vi "test-leadLag-test1.vi"(8 "error in (no error)":errorcluster) -> (0 "error out":errorcluster, 3 "All  PASSED":bool)   [LabVIEW 2019]
uses:
  <vilib>/Rock Robotics/WPI/ThirdParty/JAS_Junk/TrajLib/Util_GetTime.vi
  <vilib>/Rock Robotics/WPI/ThirdParty/JAS_Junk/TrajLib/Trajectory_Library.lvlib
panel:
  out "Lag Test Passed 2":bool
  out "Lag Chart 2":cluster{"Output":dbl, dbl}(graph)
  out "Lead Lag Test Passed":bool
  out "Lead Lag Chart":cluster{"Output":dbl, dbl}(graph)
  out "Lead Test Passed":bool
  out "Lead Test Chart":cluster{"Output":dbl, dbl}(graph)
  out "Test No Lead or Lag":bool
  out "Test No Lead or Lag":cluster{"Output":dbl, dbl}(graph)
  out "Lag Test Passed":bool
  out "Lag Chart":cluster{"Output":dbl, dbl}(graph)
  # "NOT A TEST....."
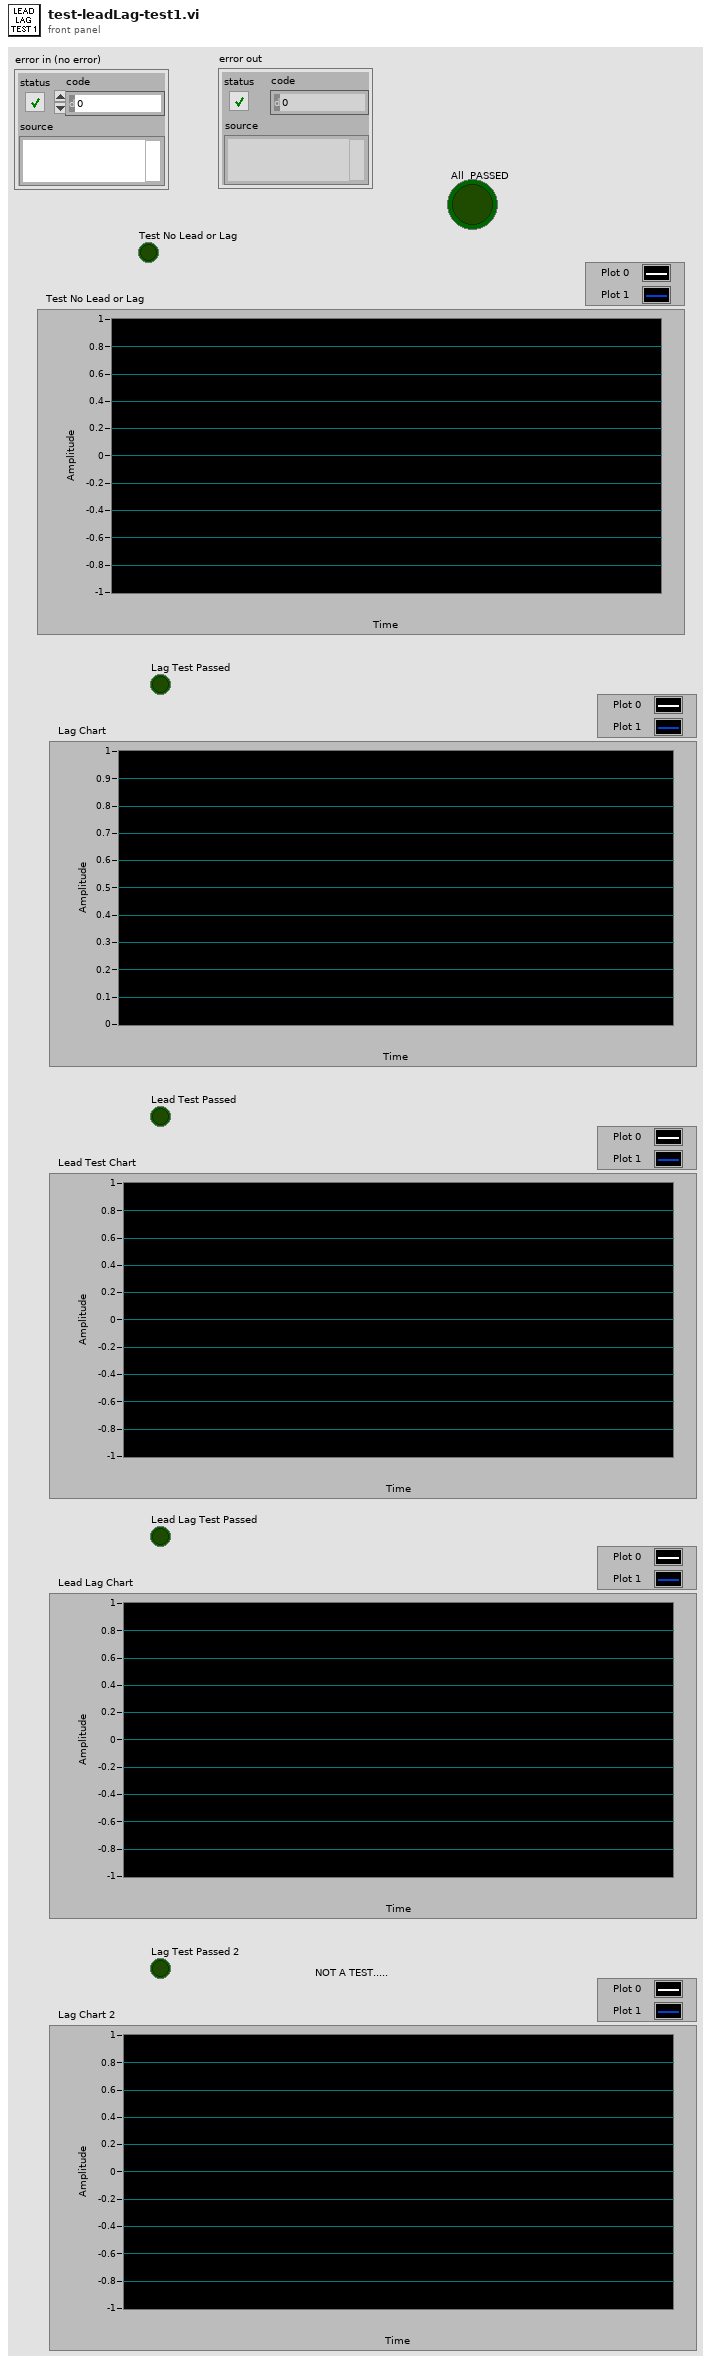
[diagram p1: front panel]
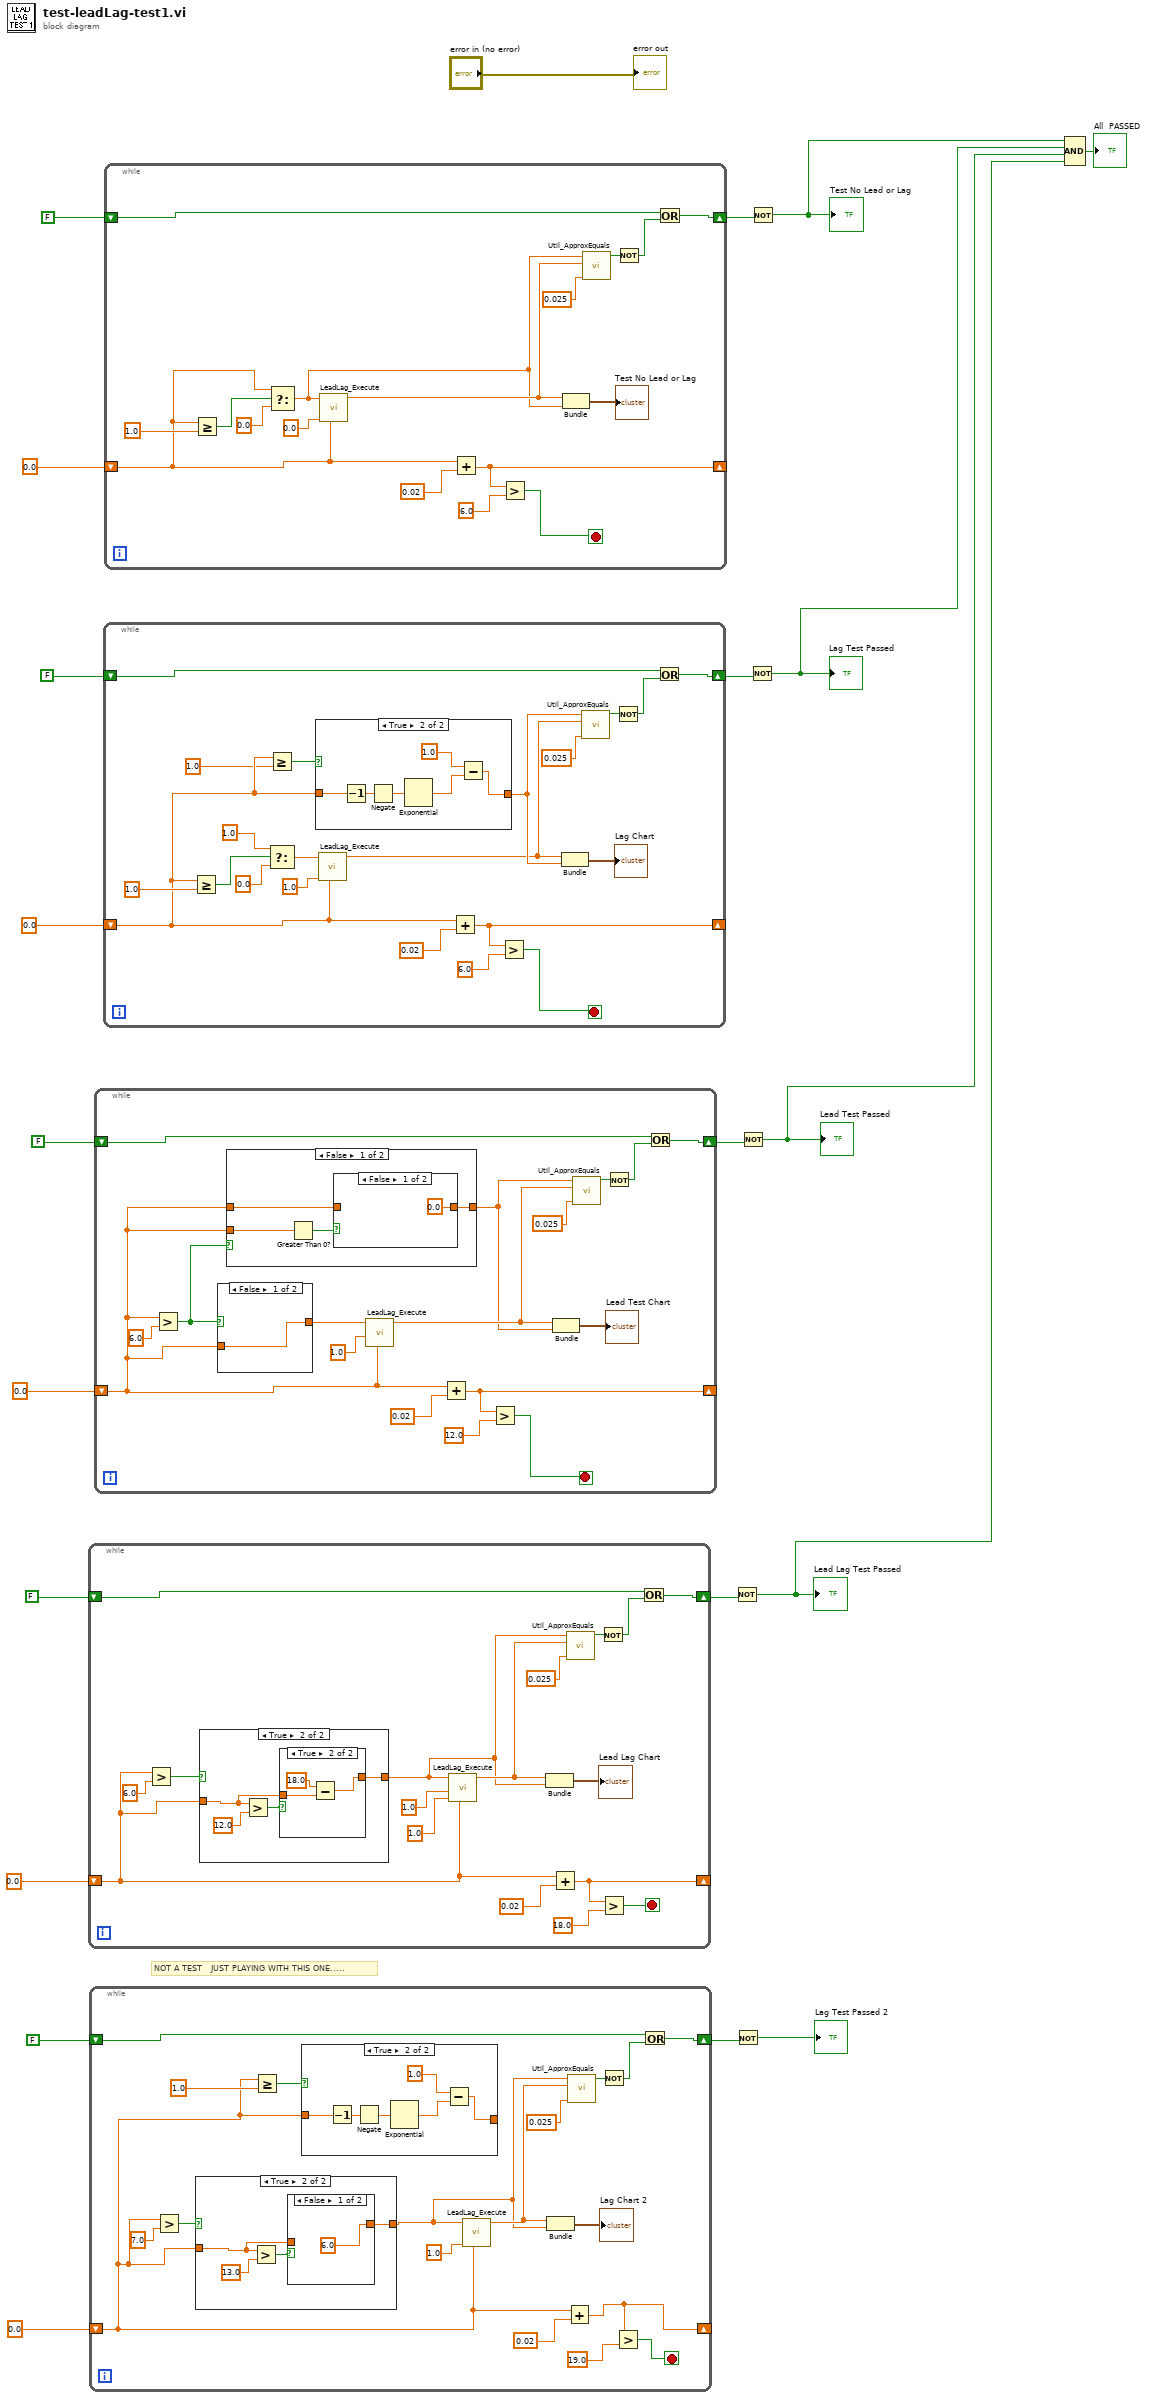
[diagram p0: block diagram]
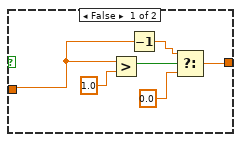
[diagram p2: hidden frame]
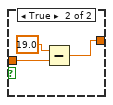
[diagram p3: hidden frame]
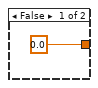
[diagram p4: hidden frame]
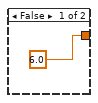
[diagram p6: hidden frame]
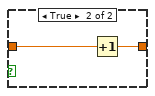
[diagram p7: hidden frame]
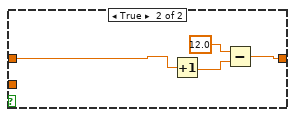
[diagram p8: hidden frame]
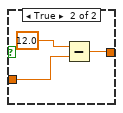
[diagram p9: hidden frame]
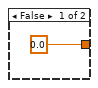
[diagram p10: hidden frame]
diagram:
  # "NOT A TEST   JUST PLAYING WITH THIS ONE....."
  n1 = while {
    shift-right: [w38] -> _
    shift-left: 0.0 -> [w27]
    shift-right: [w31] -> w11
    shift-left: FALSE -> [w33]
    stop <- w36 stop-if-true
    n2 = Greater?(x=w27, y=6.0) -> (0:w28:bool)
    n3 = case shown="True" w28 {
      tunnel: [w40 w42] -> w23
      tunnel: w27 -> [w40 w41]
      frame False {
      }
      frame True {
        n4 = Greater?(x=w41, y=12.0) -> (0:w43:bool)
        n5 = case shown="True" w43 {
          tunnel: [6.0 w48] -> w42
          tunnel: w41 -> [_ w46]
          frame False {
          }
          frame True {
            n6 = Subtract(x=18.0, y=w46) -> (x-y=w48:dbl)
          }
        }
      }
    }
    n7 = call <vilib>:"LeadLag_Execute.vi"("Time (Secs)"=w27, "Lag Time Const (Sec)"=1.0, "Lead Time Const (Sec)"=1.0 ("Lag Time Const (Sec)"), "Input"=w23) -> ("Output"=w29:dbl)  [unwired: 7 in]
    n8 = Bundle("Output"=w29, w23) -> (→"Lead Lag Chart":cluster{"Output":dbl, dbl})  [unwired: 1 in]
    n9 = Add(x=w27, y=0.02) -> (x+y=w38:dbl)
    n10 = call <vilib>:"Util_ApproxEquals.vi"("Tolerance"=0.025, "Value 2"=w29, "Value 1"=w23) -> ("ApproxEquals"=w34:bool)  [unwired: 8 in]
    n11 = Not(x=w34) -> (.not. x?=w32:bool)
    n12 = Greater?(x=w38, y=18.0) -> (0:w36:bool)
    n13 = Or(x=w33, y=w32) -> (x .or. y?=w31:bool)
  }
  n14 = while {
    shift-right: [w64] -> _
    shift-left: 0.0 -> [w50]
    shift-right: [w53] -> w8
    shift-left: FALSE -> [w55]
    stop <- w62 stop-if-true
    n15 = Greater?(x=w50, y=7.0) -> (0:w51:bool)
    n16 = case shown="True" w51 {
      tunnel: [w72 w74] -> w49
      tunnel: w50 -> [w67 w73]
      frame False {
        n17 = Greater?(x=w67, y=1.0) -> (0:w70:bool)
        n18 = Decrement(x=w67) -> (x-1=w68:dbl)
        n19 = Select(t=w68, s=w70, f=0.0) -> (s? t:f=w72:dbl)
      }
      frame True {
        n20 = Greater?(x=w73, y=13.0) -> (0:w75:bool)
        n21 = case shown="False" w75 {
          tunnel: [6.0 w80] -> w74
          tunnel: w73 -> [_ w78]
          frame False {
          }
          frame True {
            n22 = Subtract(x=19.0, y=w78) -> (x-y=w80:dbl)
          }
        }
      }
    }
    n23 = Greater Or Equal?(x=w50, y=1.0) -> (x >= y?=w61:bool)
    n24 = case shown="True" w61 {
      tunnel: w50 -> [_ w87]
      tunnel: [0.0 w82] -> _
      frame False {
      }
      frame True {
        n25 = Decrement(x=w87) -> (x-1=w85:dbl)
        n26 = Negate(x=w85) -> (-x=w84:dbl)
        n27 = Exponential(1:w84) -> (0:w83:dbl)
        n28 = Subtract(x=1.0, y=w83) -> (x-y=w82:dbl)
      }
    }
    n29 = call <vilib>:"LeadLag_Execute.vi"("Time (Secs)"=w50, "Lag Time Const (Sec)"=1.0, "Input"=w49) -> ("Output"=w58:dbl)  [unwired: 8 in]
    n30 = Bundle("Output"=w58, "f"=w49) -> (→"Lag Chart 2":cluster{"Output":dbl, "f":dbl})  [unwired: 1 in]
    n31 = Add(x=w50, y=0.02) -> (x+y=w64:dbl)
    n32 = call <vilib>:"Util_ApproxEquals.vi"("Tolerance"=0.025, "Value 2"=w58, "Value 1"=w49) -> ("ApproxEquals"=w56:bool)  [unwired: 8 in]
    n33 = Not(x=w56) -> (.not. x?=w54:bool)
    n34 = Greater?(x=w64, y=19.0) -> (0:w62:bool)
    n35 = Or(x=w55, y=w54) -> (x .or. y?=w53:bool)
  }
  n36 = while {
    shift-right: [w103] -> _
    shift-left: 0.0 -> [w88]
    shift-right: [w96] -> w14
    shift-left: FALSE -> [w98]
    stop <- w101 stop-if-true
    n37 = Greater?(x=w88, y=6.0) -> (0:w91:bool)
    n38 = case shown="False" w91 {
      tunnel: [w116 w119] -> w93
      tunnel: w88 -> [w116 w118]
      frame False {
      }
      frame True {
        n39 = Subtract(x=12.0, y=w118) -> (x-y=w119:dbl)
      }
    }
    n40 = case shown="False" w91 {
      tunnel: w88 -> [w108 w113]
      tunnel: [w107 w114] -> w90
      tunnel: w88 -> [w105 _]
      frame False {
        n41 = Greater Than 0?(x=w105) -> (x > 0?=w106:bool)
        n42 = case shown="False" w106 {
          tunnel: w108 -> [_ w111]
          tunnel: [0.0 w110] -> w107
          frame False {
          }
          frame True {
            n43 = Increment(x=w111) -> (x+1=w110:dbl)
          }
        }
      }
      frame True {
        n44 = Increment(x=w113) -> (x+1=w112:dbl)
        n45 = Subtract(x=12.0, y=w112) -> (x-y=w114:dbl)
      }
    }
    n46 = call <vilib>:"LeadLag_Execute.vi"("Time (Secs)"=w88, "Lead Time Const (Sec)"=1.0 ("Lag Time Const (Sec)"), "Input"=w93) -> ("Output"=w92:dbl)  [unwired: 8 in]
    n47 = Add(x=w88, y=0.02) -> (x+y=w103:dbl)
    n48 = Greater?(x=w103, y=12.0) -> (0:w101:bool)
    n49 = Bundle("Output"=w92, w90) -> (→"Lead Test Chart":cluster{"Output":dbl, dbl})  [unwired: 1 in]
    n50 = call <vilib>:"Util_ApproxEquals.vi"("Tolerance"=0.025, "Value 2"=w92, "Value 1"=w90) -> ("ApproxEquals"=w99:bool)  [unwired: 8 in]
    n51 = Not(x=w99) -> (.not. x?=w97:bool)
    n52 = Or(x=w98, y=w97) -> (x .or. y?=w96:bool)
  }
  n53 = while {
    shift-right: [w134] -> _
    shift-left: 0.0 -> [w128]
    shift-right: [w120] -> w20
    shift-left: FALSE -> [w122]
    stop <- w132 stop-if-true
    n54 = Greater Or Equal?(x=w128, y=1.0) -> (x >= y?=w138:bool)
    n55 = Greater Or Equal?(x=w128, y=1.0) -> (x >= y?=w131:bool)
    n56 = Select(t=1.0, s=w138, f=0.0) -> (s? t:f=w130:dbl)
    n57 = case shown="True" w131 {
      tunnel: w128 -> [_ w147]
      tunnel: [0.0 w142] -> w126
      frame False {
      }
      frame True {
        n58 = Decrement(x=w147) -> (x-1=w145:dbl)
        n59 = Negate(x=w145) -> (-x=w144:dbl)
        n60 = Exponential(1:w144) -> (0:w143:dbl)
        n61 = Subtract(x=1.0, y=w143) -> (x-y=w142:dbl)
      }
    }
    n62 = call <vilib>:"LeadLag_Execute.vi"("Time (Secs)"=w128, "Lag Time Const (Sec)"=1.0, "Input"=w130) -> ("Output"=w125:dbl)  [unwired: 8 in]
    n63 = Add(x=w128, y=0.02) -> (x+y=w134:dbl)
    n64 = Greater?(x=w134, y=6.0) -> (0:w132:bool)
    n65 = Bundle("Output"=w125, w126) -> (→"Lag Chart":cluster{"Output":dbl, dbl})  [unwired: 1 in]
    n66 = call <vilib>:"Util_ApproxEquals.vi"("Tolerance"=0.025, "Value 2"=w125, "Value 1"=w126) -> ("ApproxEquals"=w123:bool)  [unwired: 8 in]
    n67 = Not(x=w123) -> (.not. x?=w121:bool)
    n68 = Or(x=w122, y=w121) -> (x .or. y?=w120:bool)
  }
  n69 = while {
    shift-right: [w159] -> _
    shift-left: 0.0 -> [w149]
    shift-right: [w150] -> w17
    shift-left: FALSE -> [w152]
    stop <- w157 stop-if-true
    n70 = Greater Or Equal?(x=w149, y=1.0) -> (x >= y?=w162:bool)
    n71 = Select(t=w149, s=w162, f=0.0) -> (s? t:f=w148:dbl)
    n72 = call <vilib>:"LeadLag_Execute.vi"("Time (Secs)"=w149, "Lag Time Const (Sec)"=0.0, "Input"=w148) -> ("Output"=w155:dbl)  [unwired: 8 in]
    n73 = Add(x=w149, y=0.02) -> (x+y=w159:dbl)
    n74 = Greater?(x=w159, y=6.0) -> (0:w157:bool)
    n75 = Bundle("Output"=w155, "f"=w148) -> (→"Test No Lead or Lag":cluster{"Output":dbl, "f":dbl})  [unwired: 1 in]
    n76 = call <vilib>:"Util_ApproxEquals.vi"("Tolerance"=0.025, "Value 2"=w155, "Value 1"=w148) -> ("ApproxEquals"=w153:bool)  [unwired: 8 in]
    n77 = Not(x=w153) -> (.not. x?=w151:bool)
    n78 = Or(x=w152, y=w151) -> (x .or. y?=w150:bool)
  }
  n79 = Not(x=w11) -> (.not. x?=w3:bool)
  "Lead Lag Test Passed" <- w3
  n80 = Not(x=w8) -> (.not. x?=→"Lag Test Passed 2":bool)
  n81 = Not(x=w14) -> (.not. x?=w4:bool)
  "Lead Test Passed" <- w4
  n82 = Not(x=w20) -> (.not. x?=w5:bool)
  "Lag Test Passed" <- w5
  n83 = Not(x=w17) -> (.not. x?=w6:bool)
  "Test No Lead or Lag" <- w6
  n84 = Compound Arithmetic op=AND(w6, w5, w4, w3) -> (→"All  PASSED":bool)
  "error out" <- "error in (no error)"
